vi "setScanPattern.vi"(7 "maximum frequency":dbl, 8 "error in (no error)":errorcluster, 9 "scanning mode":enum16{"triangle", "spiral"}(ring)=2, 10 "Queues":T1, 11 "scan specification - tag resonant":T2) -> (0 "error out":errorcluster, 3 "scan specification out":T2)   [LabVIEW 2010]
uses:
  scan_specification_tagResonant.ctl
  internal_queues.ctl
  line_info.ctl
  volume_with_lines.ctl
  volume_info.ctl
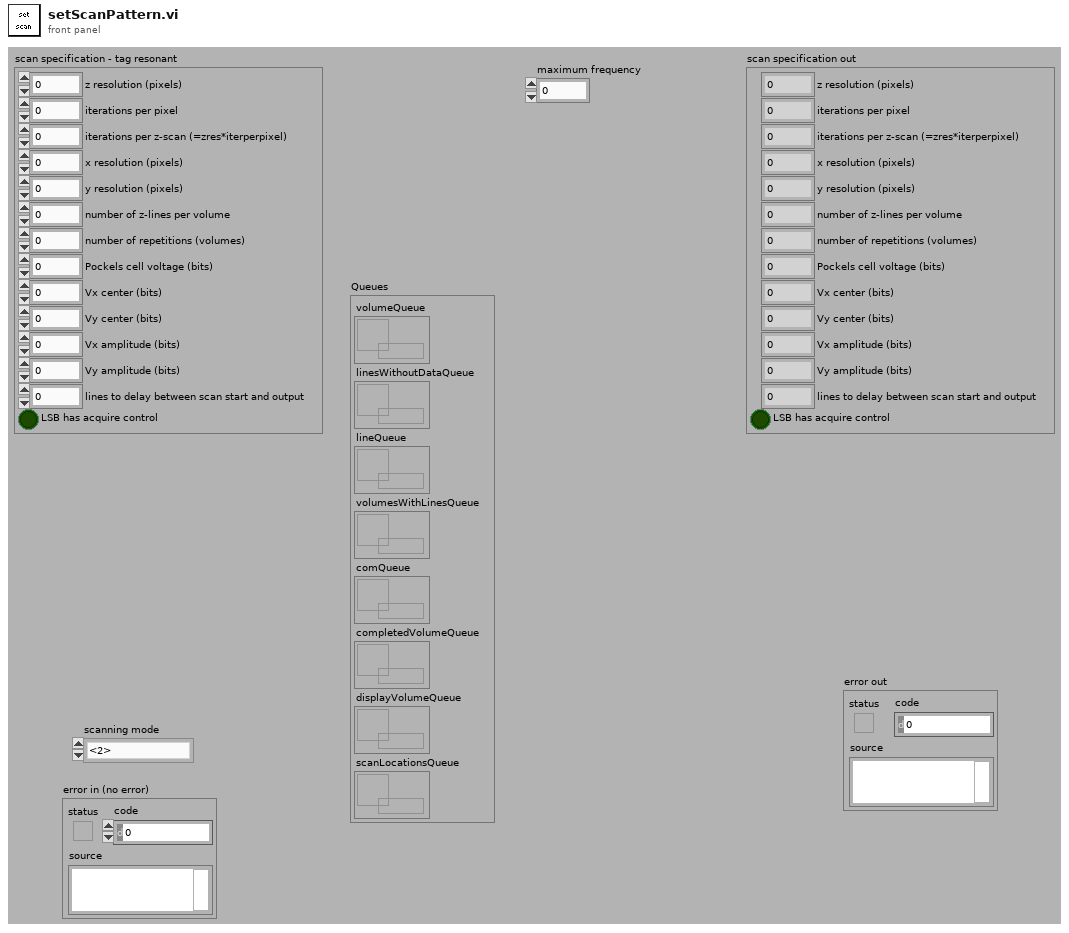
[diagram p1: front panel]
types:
  T1 = typedef "internal_queues.ctl" = cluster{"volumeQueue":refnum<queue>, "linesWithoutDataQueue":refnum<queue>, "lineQueue":refnum<queue>, "volumesWithLinesQueue":refnum<queue>, "comQueue":refnum<queue>, "completedVolumeQueue":refnum<queue>, "displayVolumeQueue":refnum<queue>, "scanLocationsQueue":refnum<queue>}
  T2 = typedef "scan_specification_tagResonant.ctl" = cluster{"z resolution (pixels)":u16, "iterations per pixel":u16, "iterations per z-scan (=zres*iterperpixel)":u16, "x resolution (pixels)":u16, "y resolution (pixels)":u16, "number of z-lines per volume":u16, "number of repetitions (volumes)":i32, "Pockels cell voltage (bits)":i16, "Vx center (bits)":i16, "Vy center (bits)":i16, "Vx amplitude (bits)":i16, "Vy amplitude (bits)":i16, "lines to delay between scan start and output":u16, "LSB has acquire control":bool}
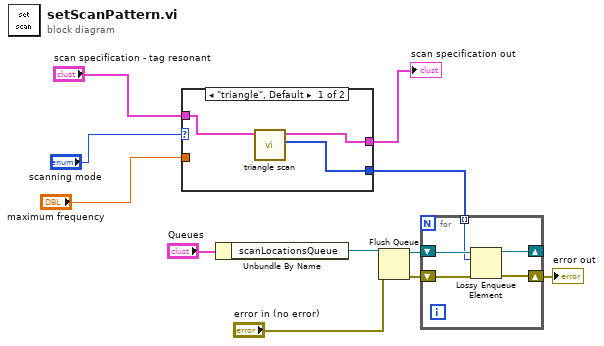
[diagram p0: block diagram]
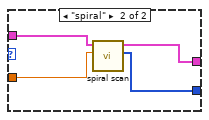
[diagram p2: hidden frame]
diagram:
  n1 = case shown="\"triangle\", Default" "scanning mode" {
    tunnel: "scan specification - tag resonant" -> [w14 w18]
    tunnel: "maximum frequency" -> [_ w17]
    tunnel: [w13 w16] -> w8
    tunnel: [w12 w15] -> w3
    frame "triangle", Default {
      n2 = call "triangle scan.vi"("scan specification"=w14) -> ("scan locations"=w12:u32[], "scan specification out"=w13:T2)  [unwired: 9 in]
    }
    frame "spiral" {
      n3 = call "spiral scan.vi"("maximum frequency"=w17, "scan specification"=w18) -> ("scan locations"=w15:u32[], "scan specification out"=w16:T2)  [unwired: 8 in]
    }
  }
  "scan specification out" <- w8
  n4 = Unbundle By Name("Queues") -> ("scanLocationsQueue"=w6:refnum<queue>)
  n5 = Flush Queue(queue=w6, error in (no error)="error in (no error)") -> (queue out=w4:refnum<queue>, error out=w5:errorcluster)  [unwired: 1 out]
  n6 = for {
    shift-right: [w22] -> w1
    shift-left: w5 -> [w23]
    shift-right: [w20] -> _
    shift-left: w4 -> [w21]
    tunnel: w3 -> [w19] mode=indexing
    n7 = Lossy Enqueue Element(queue=w21, element=w19, error in (no error)=w23) -> (queue out=w20:refnum<queue>, error out=w22:errorcluster)  [unwired: 2 out]
  }
  "error out" <- w1
